vi "Close.vi"(8 "error in (no error)":errorcluster, 11 "ArduinoAIReal in":refnum<class "Arduino.lvclass">) -> (0 "error out":errorcluster)   [LabVIEW 2020, in "Arduino.lvlib" / "Arduino.lvclass"]
doc: "- closes arduino comunication"
uses:
  Arduino.lvclass
  Arduino.lvclass/Arduino.ctl
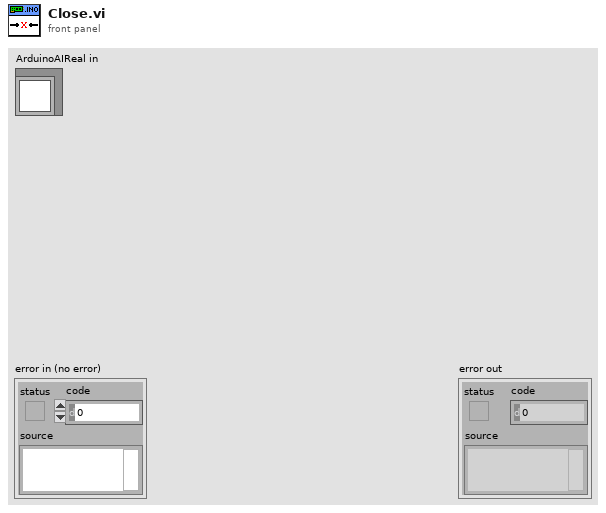
[diagram p1: front panel]
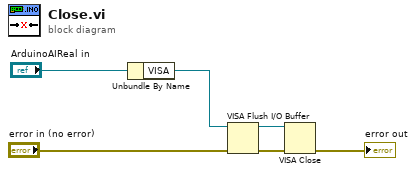
[diagram p0: block diagram]
diagram:
  n1 = Unbundle By Name("ArduinoAIReal in") -> ("VISA"=w1:refnum<visa-resource-name>)
  n2 = VISA Flush I/O Buffer(VISA resource name=w1, error in (no error)="error in (no error)") -> (VISA resource name out=w3:refnum<visa-resource-name>, error out=w2:errorcluster)  [unwired: 1 in]
  n3 = VISA Close(VISA resource name=w3, error in (no error)=w2) -> (error out=→"error out":errorcluster)
